vi "oven_switch.vi"() -> (0 "Final state":bool)   [LabVIEW 2012]
uses:
  oven_state_global.vi
panel:
  out "Previous state":bool
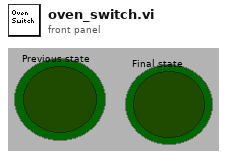
[diagram p1: front panel]
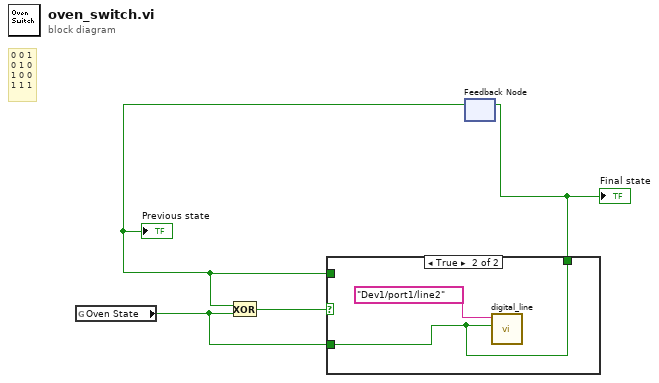
[diagram p0: block diagram]
diagram:
  # "0 0 1\n0 1 0\n1 0 0\n1 1 1"
  n1 = global read "oven_state_global.vi" "Oven State"() -> (w1:bool)
  n2 = feedback #1() -> (w3:bool)  [unwired: 1 in]
  "Previous state" <- w3
  n3 = Exclusive Or(1:w1, 2:w3) -> (0:w2:bool)
  n4 = case shown="True" w2 {
    tunnel: [w5 w6] -> w4
    tunnel: w1 -> [_ w6]
    tunnel: w3 -> [w5 _]
    frame False {
    }
    frame True {
      n5 = call "digital_line.vi"("NewVal"=w6, "lines"=tag "Dev1/port1/line2") -> ()  [unwired: 2 in]
    }
  }
  "Final state" <- w4
  n6 = feedback-in #1(w4) -> ()
